vi "global variables.vi"() -> ()   [LabVIEW 2021]
panel:
  in  "cam and 2p status logfile format":string
  in  "valid DAQmx device []":string[](array[string])=["Dev1-USB6259", "SimDev2-USB6259"]
  in  "stim logfile format":string="%15s, %15s"
  in  "log float precision":i16=8
  in  "system logs subdir":string="system-control-logs"
  in  "port position char":string[](array[string])=["L", "M", "R"]
  in  "sensirion subdir":string="sensirion-arduino-logs"
  in  "default data directory":path=path "D:/c_swain/zf_correlative_microscopy/raw_data"
  in  "stim config subdir":string="stim-configs"
  in  "odor-manifold config subdir":string="odor-manifold-configs"
  in  "binary file name":string="Binary Data File"
  in  "binary file pattern":string="*.bin"
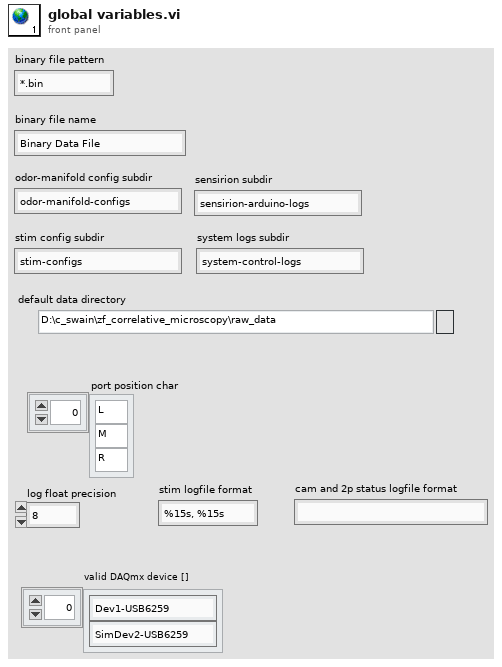
[diagram p1: front panel]
diagram:
